vi "Get Data.vi"(11 "VISA Input":refnum<visa-resource-name>) -> (0 "String":string, 1 "X10~X17":bool[](array[boolean]), 2 "X0~X7":bool[](array[boolean]), 3 "VISA Output":refnum<visa-resource-name>)   [LabVIEW 2009]
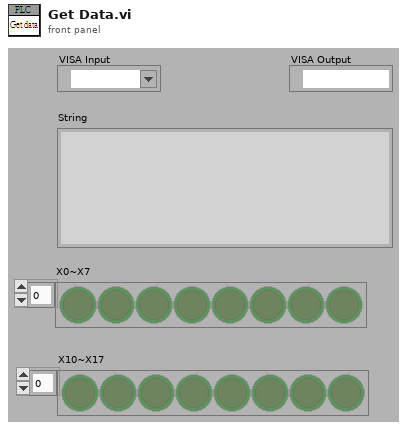
[diagram p1: front panel]
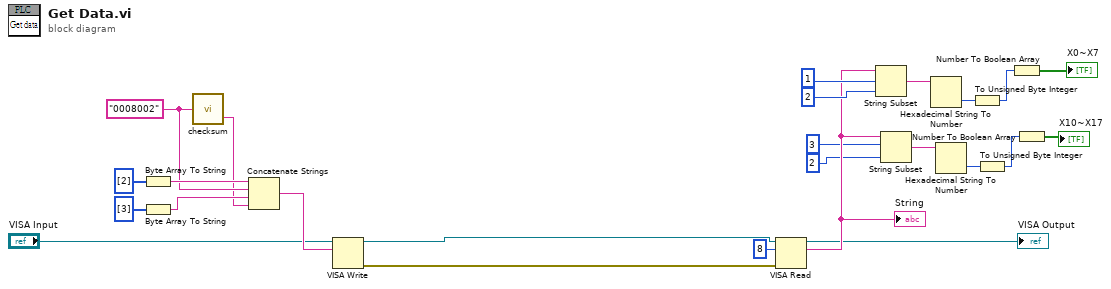
[diagram p0: block diagram]
diagram:
  w21 = "0008002"
  n1 = Byte Array To String(unsigned byte array=u8[] [2]) -> (string=w23:string)
  n2 = Byte Array To String(unsigned byte array=u8[] [3]) -> (string=w22:string)
  n3 = call "checksum.vi"("Data"=w21) -> ("Check Sum"=w20:string)  [unwired: 2 in, 1 out]
  n4 = Concatenate Strings(w23, w21, w22, w20) -> (w19:string)
  n5 = VISA Write(VISA resource name="VISA Input", write buffer=w19) -> (VISA resource name out=w3:refnum<visa-resource-name>, error out=w2:errorcluster)  [unwired: 1 in, 1 out]
  n6 = VISA Read(VISA resource name=w3, byte count=u32 8, error in (no error)=w2) -> (VISA resource name out=→"VISA Output":refnum<visa-resource-name>, read buffer=w9:string)  [unwired: 2 out]
  "String" <- w9
  n7 = String Subset(string=w9, offset (0)=1, length (rest)=2 ("length (rest)")) -> (substring=w15:string)
  n8 = String Subset(string=w9, offset (0)=3, length (rest)=2 ("length (rest)")) -> (substring=w10:string)
  n9 = Hexadecimal String To Number(string=w15) -> (number=w14:u32)  [unwired: 2 in, 1 out]
  n10 = Hexadecimal String To Number(string=w10) -> (number=w11:u32)  [unwired: 2 in, 1 out]
  n11 = To Unsigned Byte Integer(number=w14) -> (unsigned 8bit integer=w13:u8)
  n12 = To Unsigned Byte Integer(number=w11) -> (unsigned 8bit integer=w12:u8)
  n13 = Number To Boolean Array(number=w13) -> (Boolean array=→"X0~X7":bool[])
  n14 = Number To Boolean Array(number=w12) -> (Boolean array=→"X10~X17":bool[])
